vi "Calculate Buffer Index for Label Data (AIM_AIT).vi"(9 "Iteration":i32) -> (1 "Buffer index":u32)   [LabVIEW 2015, in "AIT 429 Engine.lvlib"]
uses:
  AIT 429 Engine.lvlib
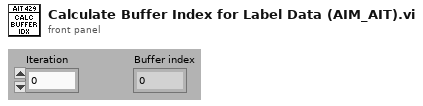
[diagram p1: front panel]
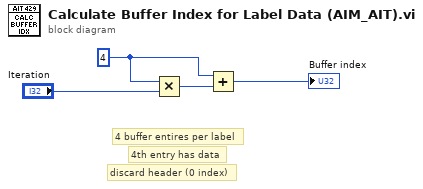
[diagram p0: block diagram]
diagram:
  w1 = u32 4 ("x")
  # "4 buffer entires per label"
  # "discard header (0 index)"
  # "4th entry has data"
  n1 = Multiply(x=w1, y="Iteration") -> (x*y=w3:u32)
  n2 = Add(x=w1, y=w3) -> (x+y=→"Buffer index":u32)
